vi "Get Toolkit Used List.vi"(10 "Version":string, 11 "Exe License Path":path) -> (0 "error out":errorcluster, 3 "Open Source Toolkit Used":string[](array[string]))   [LabVIEW 2020]
uses:
  <userlib>/_OpenG.lib/lvzip/lvzip.llb/ZLIB Open Unzip Archive__ogtk.vi
  <userlib>/_OpenG.lib/lvzip/lvzip.llb/ZLIB Extract File__ogtk.vi
  <vilib>/JKI/VIPM API/VIPM API_vipm_api.lvlib
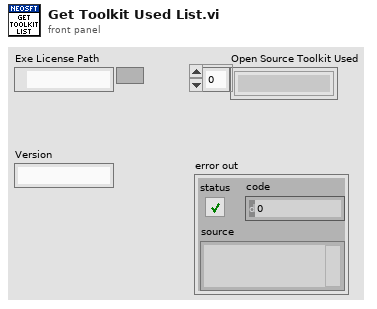
[diagram p1: front panel]
types:
  T1 = typedef "VIPM API_vipm_api.lvlib/Library Contents Cluster_vipm_api.ctl" = cluster{"Package Name":string, "Version":string, "Display Name":string, "Repository Name":string, "Company Name":string, "License Type":string, "Installed":bool, "Deprecated":bool, "Dependency or Conflict Problem":bool, "Downloaded":bool}
  T2 = typedef "ZLIB Unzip Handle__ogtk.ctl" = refnum<k1>
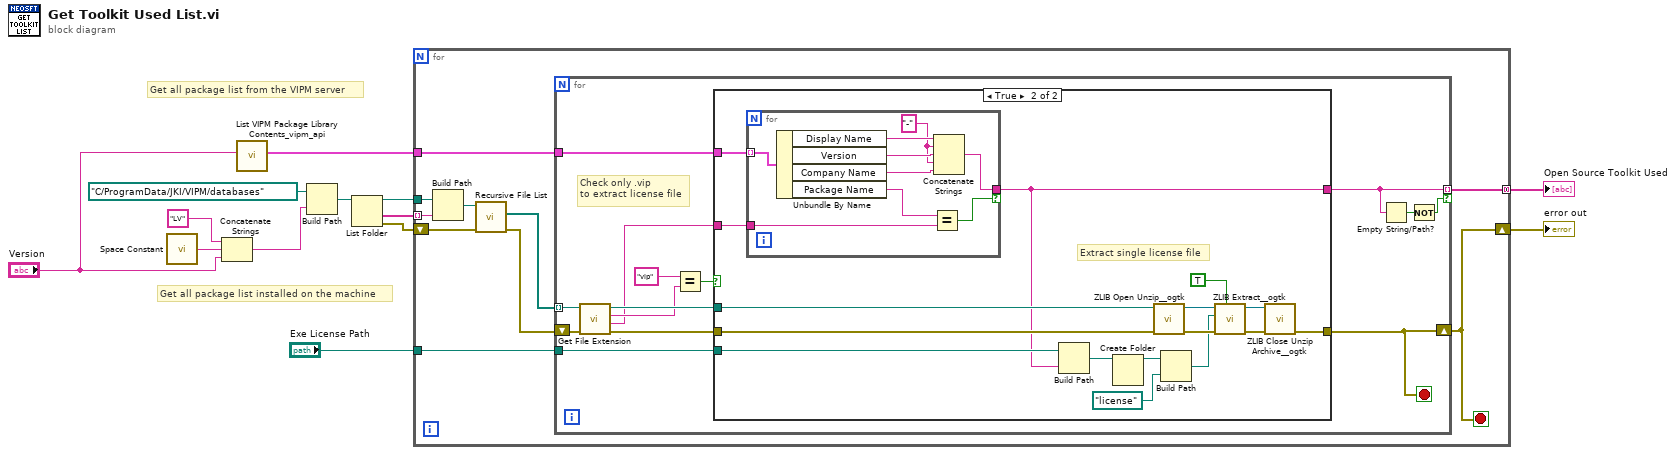
[diagram p0: block diagram]
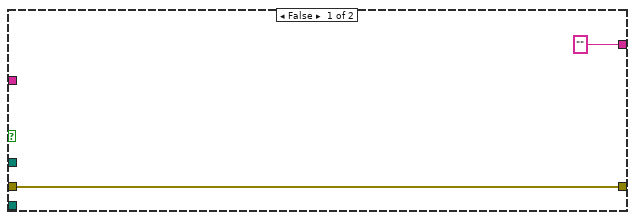
[diagram p2: hidden frame]
diagram:
  # "Get all package list from the VIPM server"
  # "Get all package list installed on the machine"
  n1 = call <vilib>:"Space Constant.vi"() -> ("String"=w5:string)
  n2 = Concatenate Strings("LV" ("string"), w5, "Version") -> (w3:string)
  n3 = call <vilib>:"List VIPM Package Library Contents_vipm_api.vi"("LabVIEW Version"="Version") -> ("Library Contents []"=w12:T1[])  [unwired: 8 in, 2 out]
  n4 = Build Path(base path=path "C:/ProgramData/JKI/VIPM/databases", name or relative path=w3) -> (appended path=w6:path)
  n5 = List Folder(path=w6) -> (path out=w7:path, folder names=w8:string[], error out=w9:errorcluster)  [unwired: 3 in, 1 out]
  n6 = for {
    tunnel: w7 -> [w23]
    tunnel: w8 -> [w22] mode=indexing
    shift-right: [w17] -> w1
    shift-left: w9 -> [w19]
    tunnel: "Exe License Path" -> [w16]
    tunnel: w12 -> [w15]
    tunnel: [w14] -> w13 mode=concatenating
    stop <- w17 stop-if-true
    n7 = Build Path(base path=w23, name or relative path=w22) -> (appended path=w21:path)
    n8 = call <vilib>:"Recursive File List.vi"("error in (no error)"=w19, "Folder Path"=w21) -> ("error out"=w18:errorcluster, "All Files in Dir"=w20:path[])  [unwired: 5 in, 3 out]
    n9 = for {
      tunnel: w20 -> [w37] mode=indexing
      shift-right: [w32] -> w17
      shift-left: w18 -> [w34]
      tunnel: w16 -> [w24]
      tunnel: w15 -> [w29]
      tunnel: [w27] -> w14 mode=indexing if=w25
      stop <- w32 stop-if-true
      # "Check only .vip\nto extract license file"
      n10 = call <vilib>:"Get File Extension.vi"("error in (no error)"=w34, "file"=w37) -> ("error out"=w33:errorcluster, "filename without extension"=w28:string, "lowercase file extension"=w30:string, "dup file"=w35:path)  [unwired: 5 in, 1 out]
      n11 = Equal?(x="vip" ("y"), y=w30) -> (x = y?=w36:bool)
      n12 = case shown="True" w36 {
        tunnel: w35 -> [_ w55]
        tunnel: w33 -> [w39 w52]
        tunnel: [w39 w51] -> w32
        tunnel: w29 -> [_ w44]
        tunnel: w28 -> [_ w43]
        tunnel: ["" ("Display Name") w40] -> w27
        tunnel: w24 -> [_ w42]
        frame False {
        }
        frame True {
          # "Extract single license file"
          n13 = for {
            tunnel: w44 -> [w64] mode=indexing
            tunnel: w43 -> [w63]
            tunnel: [w56] -> w40 if=w62
            w58 = "-"
            n14 = Unbundle By Name(w64) -> ("Display Name"=w60:string, "Version"=w59:string, "Company Name"=w57:string, "Package Name"=w61:string)
            n15 = Equal?(x=w61, y=w63) -> (x = y?=w62:bool)
            n16 = Concatenate Strings(w60, w58, w59, w58, w57) -> (w56:string)
          }
          n17 = Build Path(base path=w42, name or relative path=w40) -> (appended path=w41:path)
          n18 = Create Folder(path (use dialog)=w41) -> (created path=w45:path)  [unwired: 2 in, 2 out]
          n19 = call-poly <userlib>:"ZLIB Open Unzip__ogtk.vi"("error in (no error)"=w52, "archive name"=w55) -> ("error out"=w49:errorcluster, "unzip Refnum"=w48:T2)  [unwired: 4 in]
          n20 = Build Path(base path=w45, name or relative path=path "license") -> (appended path=w46:path)
          n21 = call-poly <userlib>:"ZLIB Extract__ogtk.vi"("overwrite (F)"=TRUE, "error in (no error)"=w49, "target path"=w46, "unzip Refnum"=w48) -> ("error out"=w53:errorcluster, "unzip Refnum out"=w54:T2)  [unwired: 4 in]
          n22 = call <userlib>:"ZLIB Close Unzip Archive__ogtk.vi"("error in (no error)"=w53, "unzip Refnum"=w54) -> ("error out"=w51:errorcluster)  [unwired: 5 in]
        }
      }
      n23 = Empty String/Path?(string/path=w27) -> (empty?=w26:bool)
      n24 = Not(x=w26) -> (.not. x?=w25:bool)
    }
  }
  "Open Source Toolkit Used" <- w13
  "error out" <- w1
